vi "XYConstantCurr.vi"() -> ()   [LabVIEW 2014]
uses:
  <vilib>/Native 3D Graph/xcontrol/3DPC_SurfacePlot.xctl
  <vilib>/Instr/_visa.llb/VISA Configure Serial Port (Instr).vi
panel:
  out "XZ Graph":cluster{dbl[], dbl[]}(graph)
  in  "ScanStop":bool
  in  "STM Modefier":bool
  in  "LimitBeyondNum":i32
  out "Counting":i32(graph)
  out "ApprStop?":bool
  out "ZValue":dbl[](array[numeric])
  out "ProcRefCurr":dbl
  out "RMOVERR?":string
  out "XYPOS":cluster{dbl[], dbl[]}(graph)
  out "PIZPOSDia":dbl(graph)
  in  "ApproachStop":bool
  out "PIZERR? 2":string
  out "PIZERR?":string
  out "PreCurrDia":dbl(graph)
  out "3D Graph":refnum<class "Base Datatype.lvclass">[](xcontrol)
  in  "Y init/um":dbl format="%#_13g"
  in  "X init/um":dbl format="%#_13g"
  out "RefCurr":dbl
  out "PresCurr":dbl
  in  "PointNumToFresRefCurr":i32
  in  "ColumnNum":i32
  in  "RowNum":i32
  in  "ProbeBrokenDownToRefCurr %":dbl
  in  "TolerantIntervalToRefCurr %":dbl
  in  "CurrDecline %":dbl
  in  "PIZApproachStep/um":dbl
  in  "PIZAdjustStep/um":dbl
  in  "RoughYStep/um":dbl
  in  "RoughXStep/um":dbl
  out "PIZPos":dbl
  out "RoughZPos":dbl
  out "RoughYPos":dbl
  out "RoughXPos":dbl
  out "Outleak":string
  in  "PIZ":refnum<visa-resource-name>
  in  "RoughXYZ":refnum<visa-resource-name>
  in  "Volt":refnum<visa-resource-name>
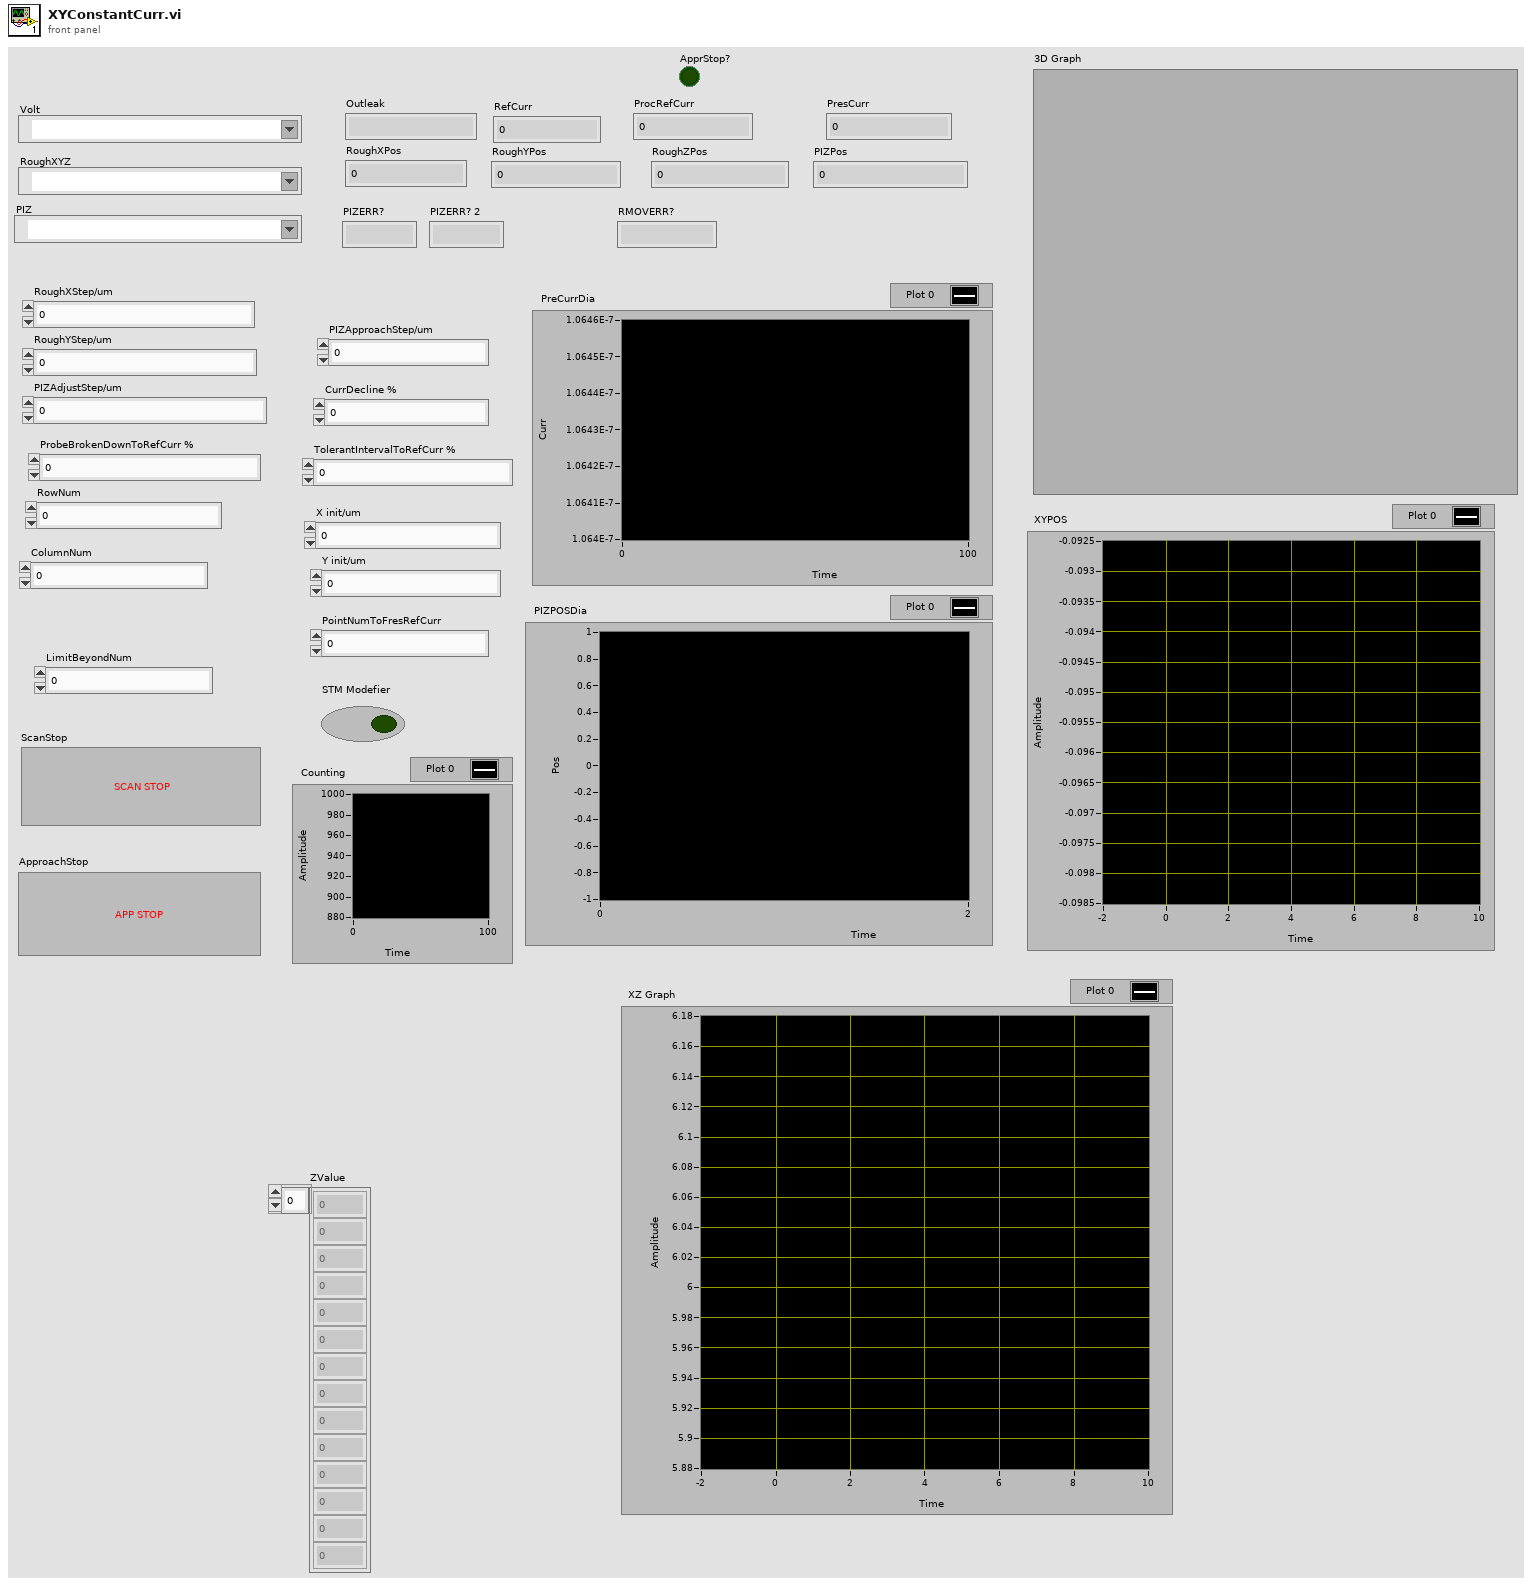
[diagram p1: front panel]
types:
  T1 = typedef "NI_Matrix.lvlib/RealMatrix.ctl" = dbl[][]
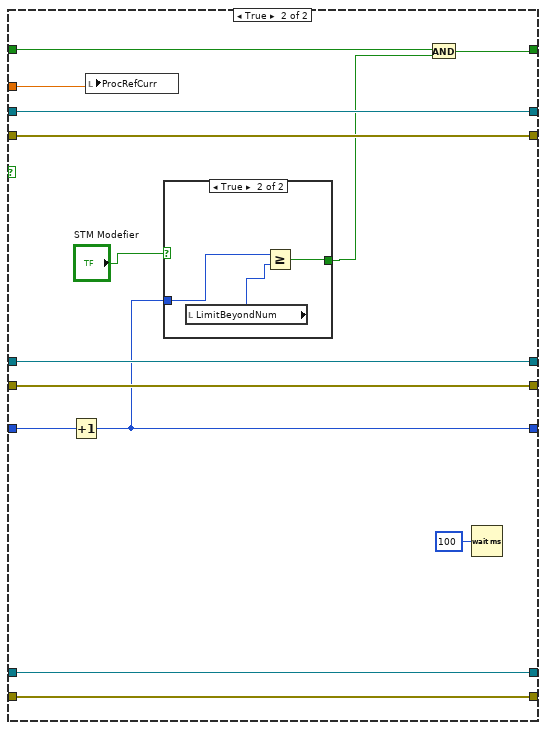
[diagram p2: hidden frame]
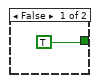
[diagram p3: hidden frame]
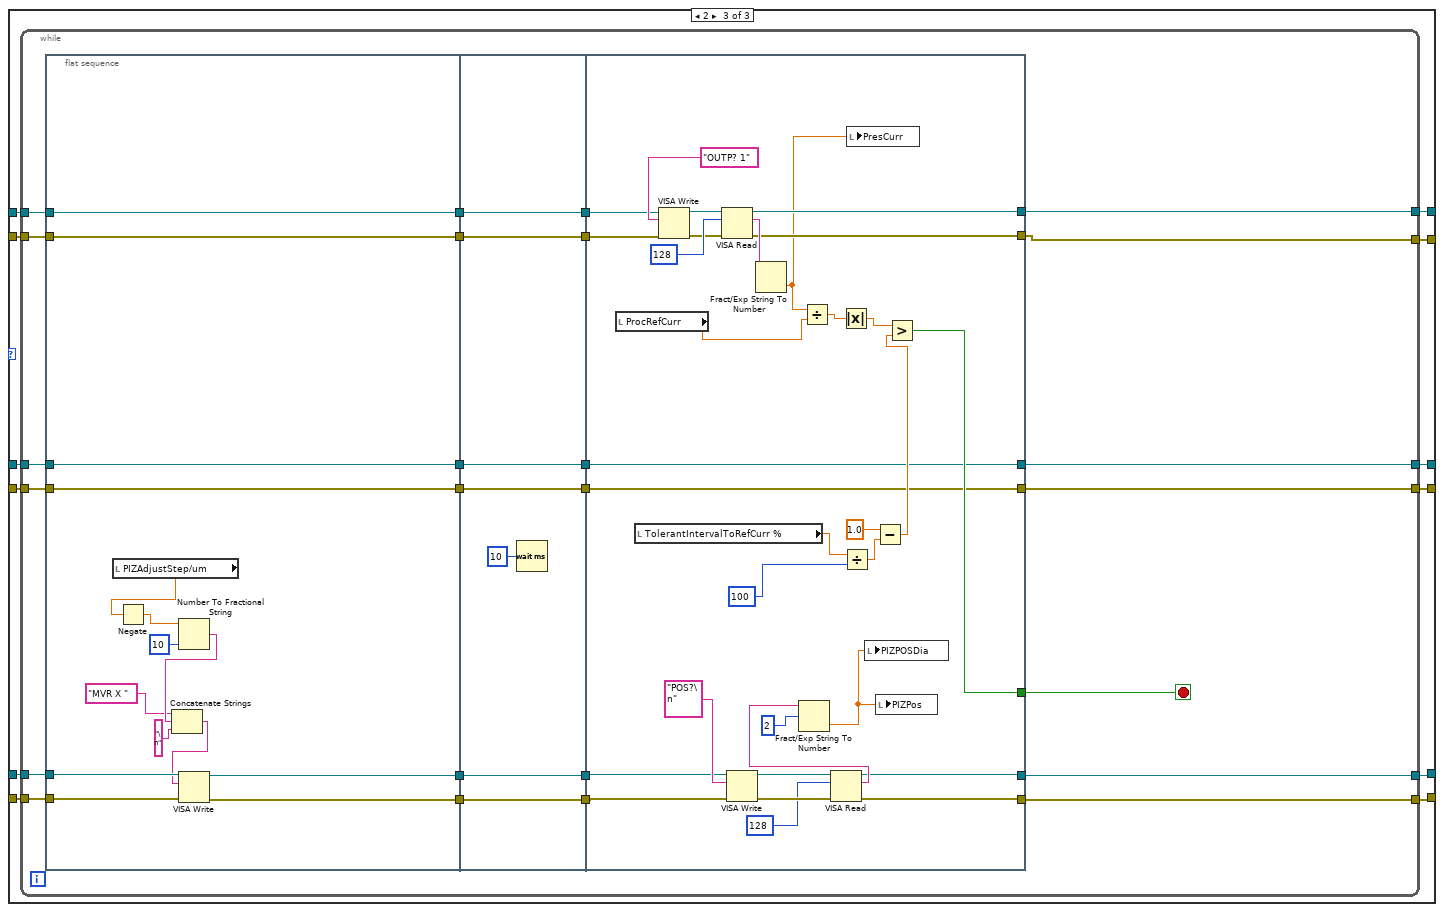
[diagram p5: hidden frame]
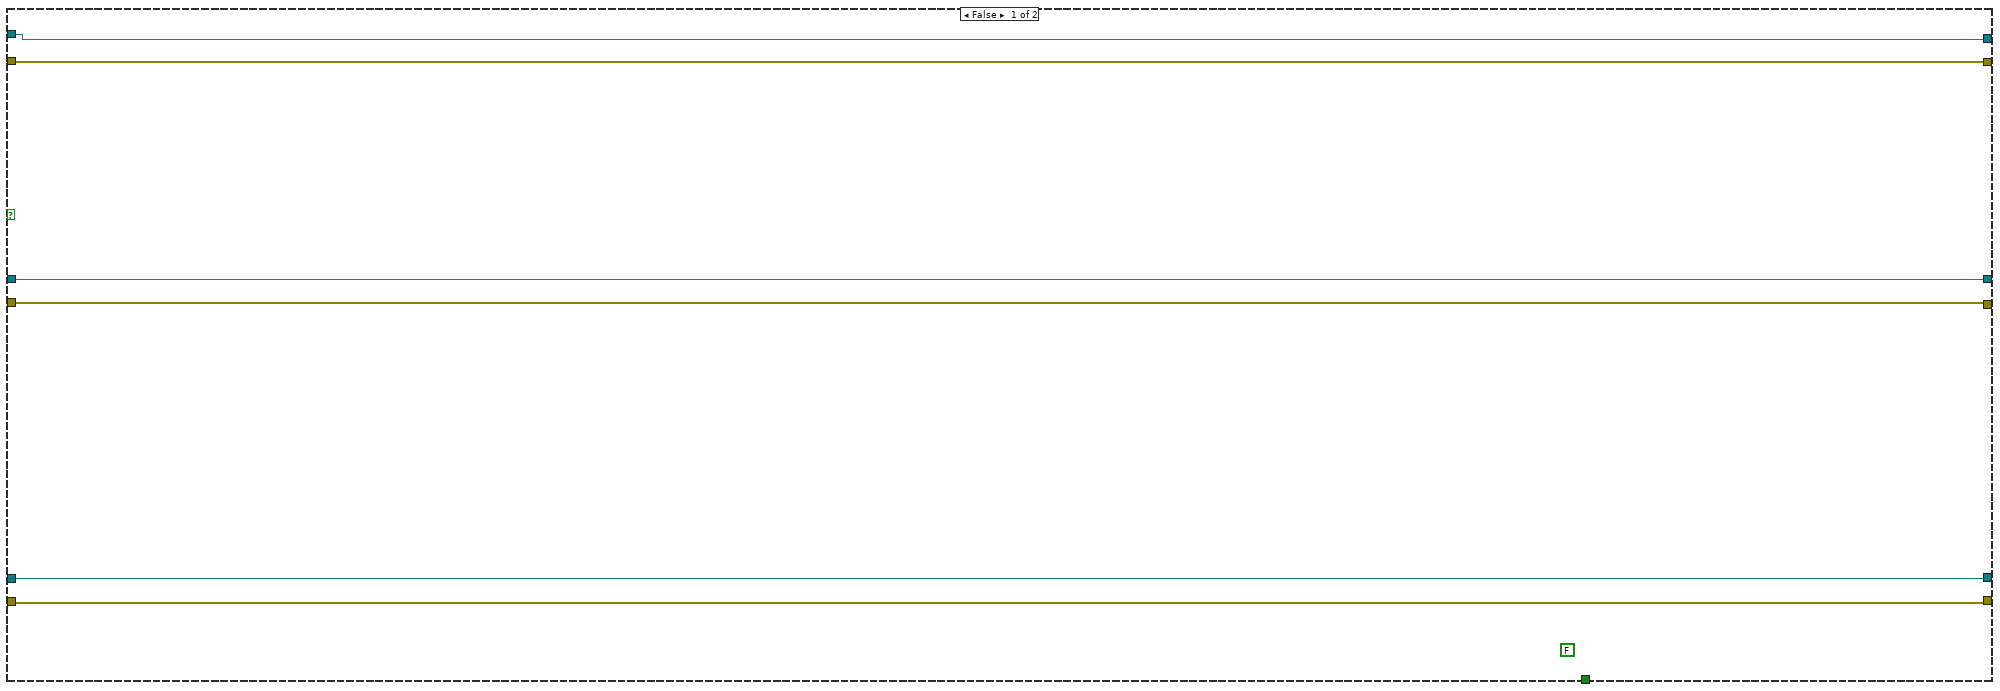
[diagram p6: hidden frame]
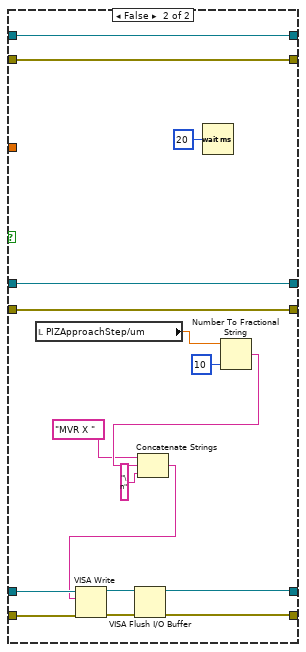
[diagram p8: hidden frame]
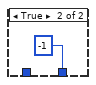
[diagram p10: hidden frame]
diagram:
  n1 = flat-sequence {
    tunnel: [w120] -> w82
    tunnel: [w119] -> w81
    tunnel: [w118] -> w80
    tunnel: [w117] -> w79
    tunnel: [w115] -> w78
    tunnel: [w114] -> w77
    tunnel: w82 -> [w185]
    tunnel: w81 -> [w184]
    tunnel: w80 -> [w169]
    tunnel: w79 -> [w168]
    tunnel: w78 -> [w193]
    tunnel: w77 -> [w192]
    tunnel: [w140] -> w76
    tunnel: [w139] -> w75
    tunnel: [w173] -> w74
    tunnel: [w172] -> w73
    tunnel: [w130] -> w72
    tunnel: [w129] -> w71
    tunnel: [w138] -> w66
    tunnel: w76 -> [w199]
    tunnel: w75 -> [w198]
    tunnel: w74 -> [w204]
    tunnel: w73 -> [w203]
    tunnel: w72 -> [w202]
    tunnel: w71 -> [w201]
    tunnel: [w204] -> w70
    tunnel: [w203] -> w69
    tunnel: [w202] -> w68
    tunnel: [w201] -> w67
    tunnel: w66 -> [w197]
    tunnel: [w194] -> w65
    tunnel: [w196] -> w64
    tunnel: [w195] -> w63
    tunnel: w70 -> [w232]
    tunnel: w69 -> [w231]
    tunnel: w68 -> [w230]
    tunnel: w67 -> [w229]
    tunnel: w65 -> [w221]
    tunnel: w64 -> [w234]
    tunnel: w63 -> [w233]
    tunnel: [w227] -> w6
    tunnel: [w226] -> w8
    tunnel: [w225] -> w10
    tunnel: [w224] -> w12
    tunnel: [w223] -> w14
    tunnel: [w222] -> w16
    tunnel: w16 -> [w320]
    tunnel: [w320] -> w15
    tunnel: w14 -> [w319]
    tunnel: [w319] -> w13
    tunnel: w12 -> [w318]
    tunnel: [w318] -> w11
    tunnel: w10 -> [w317]
    tunnel: [w317] -> w9
    tunnel: w8 -> [w316]
    tunnel: [w316] -> w7
    tunnel: w6 -> [w315]
    tunnel: [w315] -> w5
    tunnel: w15 -> [w335]
    tunnel: w13 -> [w336]
    tunnel: w11 -> [w323]
    tunnel: w9 -> [w324]
    tunnel: w7 -> [w349]
    tunnel: w5 -> [w350]
    tunnel: [w347] -> w62
    tunnel: [w346] -> w61
    tunnel: [w345] -> w60
    tunnel: [w344] -> w59
    tunnel: [w343] -> w58
    tunnel: [w342] -> w57
    tunnel: [w341] -> w39
    tunnel: [w340] -> w38
    tunnel: [w339] -> w37
    tunnel: w62 -> [w1192]
    tunnel: w61 -> [w1191]
    tunnel: w60 -> [w1194]
    tunnel: w59 -> [w1193]
    tunnel: w58 -> [w1199]
    tunnel: w57 -> [w1198]
    tunnel: [w1197] -> w56
    tunnel: [w1196] -> w55
    tunnel: [w1195] -> w54
    tunnel: [w1194] -> w53
    tunnel: [w1193] -> w52
    tunnel: [w1192] -> w51
    tunnel: [w1191] -> w50
    tunnel: w39 -> [w1189]
    tunnel: w38 -> [w1190]
    tunnel: w37 -> [w1188]
    tunnel: [w1190] -> w36
    tunnel: [w1189] -> w35
    tunnel: [w1188] -> w34
    tunnel: w56 -> [w1207]
    tunnel: w55 -> [w1206]
    tunnel: w54 -> [_]
    tunnel: w53 -> [w1214]
    tunnel: w52 -> [w1213]
    tunnel: w51 -> [w1212]
    tunnel: w50 -> [w1211]
    tunnel: [w1214] -> w49
    tunnel: [w1213] -> w48
    tunnel: [w1207] -> w47
    tunnel: [w1206] -> w46
    tunnel: [w1212] -> w45
    tunnel: [w1211] -> w44
    tunnel: w36 -> [w1210]
    tunnel: w35 -> [w1209]
    tunnel: w34 -> [w1208]
    tunnel: [w1210] -> w33
    tunnel: [w1209] -> w32
    tunnel: [w1208] -> w31
    tunnel: w49 -> [w1230]
    tunnel: w48 -> [w1229]
    tunnel: [w1220] -> w25
    tunnel: w47 -> [w1222]
    tunnel: [w1219] -> w24
    tunnel: w46 -> [w1221]
    tunnel: [w1227] -> w41
    tunnel: [w1226] -> w40
    tunnel: w45 -> [w1224]
    tunnel: w44 -> [w1223]
    tunnel: [w1224] -> w43
    tunnel: [w1223] -> w42
    tunnel: w33 -> [w1217]
    tunnel: w32 -> [w1216]
    tunnel: w31 -> [w1215]
    tunnel: [w1217] -> w29
    tunnel: [w1216] -> w28
    tunnel: [w1215] -> w27
    frame #0 {
      n2 = Wait (ms)(milliseconds to wait=u32 2000) -> ()  [unwired: 1 out]
      n3 = call-poly "VISA Configure Serial Port"("VISA resource name"="PIZ", "baud rate (9600)"=u32 115200) -> ("VISA resource name out"=w101:refnum<visa-resource-name>, "error out"=w100:errorcluster)  [unwired: 12 in]
      n4 = local write "CurrDecline %"("CurrDecline %") -> ()
      n5 = local write "TolerantIntervalToRefCurr %"("TolerantIntervalToRefCurr %") -> ()
      n6 = local write "ColumnNum"("ColumnNum") -> ()
      n7 = call-poly "VISA Configure Serial Port"("VISA resource name"="RoughXYZ", "baud rate (9600)"=u32 115200) -> ("VISA resource name out"=w92:refnum<visa-resource-name>, "error out"=w91:errorcluster)  [unwired: 12 in]
      n8 = local write "LimitBeyondNum"("LimitBeyondNum") -> ()
      n9 = local write "RowNum"("RowNum") -> ()
      n10 = local write "RoughYStep/um"("RoughYStep/um") -> ()
      n11 = local write "RoughXStep/um"("RoughXStep/um") -> ()
      n12 = local write "X init/um"("X init/um") -> ()
      n13 = VISA Write(VISA resource name=w101, write buffer="ERR?\n", error in (no error)=w100) -> (VISA resource name out=w99:refnum<visa-resource-name>, error out=w98:errorcluster)  [unwired: 1 out]
      n14 = VISA Write(VISA resource name=w92, write buffer="ERR?\n", error in (no error)=w91) -> (VISA resource name out=w89:refnum<visa-resource-name>, error out=w88:errorcluster)  [unwired: 1 out]
      n15 = VISA Read(VISA resource name=w99, byte count=u32 128, error in (no error)=w98) -> (VISA resource name out=w97:refnum<visa-resource-name>, read buffer=→"PIZERR?":string, error out=w96:errorcluster)  [unwired: 1 out]
      n16 = VISA Read(VISA resource name=w89, byte count=u32 128, error in (no error)=w88) -> (VISA resource name out=w87:refnum<visa-resource-name>, read buffer=→"RMOVERR?":string, error out=w86:errorcluster)  [unwired: 1 out]
      n17 = VISA Open(VISA resource name="Volt") -> (VISA resource name=w115:refnum<visa-resource-name>, error out=w114:errorcluster)  [unwired: 4 in]
      n18 = local write "PointNumToFresRefCurr"("PointNumToFresRefCurr") -> ()
      n19 = local write "ProbeBrokenDownToRefCurr %"("ProbeBrokenDownToRefCurr %") -> ()
      n20 = local write "PIZApproachStep/um"("PIZApproachStep/um") -> ()
      n21 = local write "PIZAdjustStep/um"("PIZAdjustStep/um") -> ()
      n22 = local write "Y init/um"("Y init/um") -> ()
      n23 = VISA Write(VISA resource name=w87, write buffer="ONL 1 1 2 1 3 1\nSVO A 1\nSVO B 1\nSVO C 1\n", error in (no error)=w86) -> (VISA resource name out=w120:refnum<visa-resource-name>, error out=w119:errorcluster)  [unwired: 1 out]
      n24 = VISA Write(VISA resource name=w97, write buffer="SVO X 1\n", error in (no error)=w96) -> (VISA resource name out=w118:refnum<visa-resource-name>, error out=w117:errorcluster)  [unwired: 1 out]
    }
    frame #1 {
      n25 = VISA Write(VISA resource name=w185, write buffer="POS? A\n", error in (no error)=w184) -> (VISA resource name out=w183:refnum<visa-resource-name>, error out=w182:errorcluster)  [unwired: 1 out]
      n26 = VISA Write(VISA resource name=w193, write buffer="OUTP? 1", error in (no error)=w192) -> (VISA resource name out=w190:refnum<visa-resource-name>, error out=w189:errorcluster)  [unwired: 1 out]
      n27 = VISA Write(VISA resource name=w169, write buffer="POS?\n", error in (no error)=w168) -> (VISA resource name out=w171:refnum<visa-resource-name>, error out=w170:errorcluster)  [unwired: 1 out]
      n28 = VISA Read(VISA resource name=w183, byte count=u32 128, error in (no error)=w182) -> (VISA resource name out=w181:refnum<visa-resource-name>, read buffer=w161:string, error out=w180:errorcluster)  [unwired: 1 out]
      n29 = VISA Read(VISA resource name=w190, byte count=u32 128, error in (no error)=w189) -> (VISA resource name out=w142:refnum<visa-resource-name>, read buffer=→"Outleak":string, error out=w141:errorcluster)  [unwired: 1 out]
      n30 = Fract/Exp String To Number(string=w161, offset=2) -> (number=→"RoughXPos":dbl)  [unwired: 2 in, 1 out]
      n31 = VISA Write(VISA resource name=w181, write buffer="POS? B\n", error in (no error)=w180) -> (VISA resource name out=w179:refnum<visa-resource-name>, error out=w178:errorcluster)  [unwired: 1 out]
      n32 = VISA Read(VISA resource name=w171, byte count=u32 128, error in (no error)=w170) -> (VISA resource name out=w132:refnum<visa-resource-name>, read buffer=w150:string, error out=w131:errorcluster)  [unwired: 1 out]
      n33 = VISA Read(VISA resource name=w179, byte count=u32 128, error in (no error)=w178) -> (VISA resource name out=w175:refnum<visa-resource-name>, read buffer=w160:string, error out=w174:errorcluster)  [unwired: 1 out]
      n34 = Fract/Exp String To Number(string=w150, offset=2) -> (number=→"PIZPos":dbl)  [unwired: 2 in, 1 out]
      n35 = Fract/Exp String To Number(string=w160, offset=2) -> (number=→"RoughYPos":dbl)  [unwired: 2 in, 1 out]
      n36 = VISA Write(VISA resource name=w132, write buffer="ERR?\n", error in (no error)=w131) -> (VISA resource name out=w137:refnum<visa-resource-name>, error out=w136:errorcluster)  [unwired: 1 out]
      n37 = VISA Write(VISA resource name=w142, write buffer="OUTP? 1", error in (no error)=w141) -> (VISA resource name out=w147:refnum<visa-resource-name>, error out=w146:errorcluster)  [unwired: 1 out]
      n38 = VISA Write(VISA resource name=w175, write buffer="POS? C\n", error in (no error)=w174) -> (VISA resource name out=w177:refnum<visa-resource-name>, error out=w176:errorcluster)  [unwired: 1 out]
      n39 = VISA Read(VISA resource name=w137, byte count=u32 128, error in (no error)=w136) -> (VISA resource name out=w130:refnum<visa-resource-name>, read buffer=→"PIZERR? 2":string, error out=w129:errorcluster)  [unwired: 1 out]
      n40 = VISA Read(VISA resource name=w177, byte count=u32 128, error in (no error)=w176) -> (VISA resource name out=w173:refnum<visa-resource-name>, read buffer=w159:string, error out=w172:errorcluster)  [unwired: 1 out]
      n41 = VISA Read(VISA resource name=w147, byte count=u32 128, error in (no error)=w146) -> (VISA resource name out=w140:refnum<visa-resource-name>, read buffer=w143:string, error out=w139:errorcluster)  [unwired: 1 out]
      n42 = Wait (ms)(milliseconds to wait=u32 1000) -> ()  [unwired: 1 out]
      n43 = Fract/Exp String To Number(string=w159, offset=2) -> (number=→"RoughZPos":dbl)  [unwired: 2 in, 1 out]
      n44 = Fract/Exp String To Number(string=w143) -> (number=w138:dbl)  [unwired: 3 in, 1 out]
      "ProcRefCurr" <- 0.0
    }
    frame #2 {
      # "Reference Curr"
      n45 = for {
        N: 50 -> [_]
        tunnel: w199 -> [w216]
        tunnel: w198 -> [w215]
        tunnel: [w213] -> w196
        tunnel: [w212] -> w195
        shift-right: [w207] -> w194
        shift-left: w197 -> [w210]
        n46 = VISA Write(VISA resource name=w216, write buffer="OUTP? 1", error in (no error)=w215) -> (VISA resource name out=w219:refnum<visa-resource-name>, error out=w218:errorcluster)  [unwired: 1 out]
        n47 = VISA Read(VISA resource name=w219, byte count=u32 128, error in (no error)=w218) -> (VISA resource name out=w213:refnum<visa-resource-name>, read buffer=w211:string, error out=w212:errorcluster)  [unwired: 1 out]
        n48 = Wait (ms)(milliseconds to wait=u32 1) -> ()  [unwired: 1 out]
        n49 = Fract/Exp String To Number(string=w211) -> (number=w205:dbl)  [unwired: 3 in, 1 out]
        "PresCurr" <- w205
        n50 = Add(x=w205, y=w210) -> (x+y=w209:dbl)
        n51 = Divide(x=w209, y=2.0) -> (x/y=w207:dbl)
      }
      "RefCurr" <- w194
    }
    frame #3 {
      n52 = local read "PIZApproachStep/um"() -> (w228:dbl)
      n53 = Divide(x=30.0, y=w228) -> (x/y=w236:dbl)
      n54 = Round Toward -Infinity(1:w236) -> (0:w235:dbl)
      n55 = for {
        N: w235 -> [_]
        tunnel: w234 -> [w274]
        tunnel: w233 -> [w273]
        tunnel: w232 -> [w270]
        tunnel: w231 -> [w269]
        tunnel: w230 -> [w255]
        tunnel: w229 -> [w254]
        tunnel: [w266] -> w227
        tunnel: [w265] -> w226
        tunnel: [w264] -> w225
        tunnel: [w263] -> w224
        tunnel: [w262] -> w223
        tunnel: [w261] -> w222
        tunnel: w221 -> [w250]
        shift-right: [w238] -> _
        shift-left: 0 -> [w239]
        stop <- w241 stop-if-true
        n56 = VISA Write(VISA resource name=w274, write buffer="OUTP? 1", error in (no error)=w273) -> (VISA resource name out=w279:refnum<visa-resource-name>, error out=w278:errorcluster)  [unwired: 1 out]
        n57 = VISA Write(VISA resource name=w255, write buffer="POS?\n", error in (no error)=w254) -> (VISA resource name out=w260:refnum<visa-resource-name>, error out=w259:errorcluster)  [unwired: 1 out]
        n58 = VISA Read(VISA resource name=w279, byte count=u32 128, error in (no error)=w278) -> (VISA resource name out=w272:refnum<visa-resource-name>, read buffer=w275:string, error out=w271:errorcluster)  [unwired: 1 out]
        n59 = VISA Read(VISA resource name=w260, byte count=u32 128, error in (no error)=w259) -> (VISA resource name out=w253:refnum<visa-resource-name>, read buffer=w256:string, error out=w252:errorcluster)  [unwired: 1 out]
        n60 = Fract/Exp String To Number(string=w275) -> (number=w240:dbl)  [unwired: 3 in, 1 out]
        "PreCurrDia" <- w240
        n61 = local read "CurrDecline %"() -> (w245:dbl)
        n62 = Fract/Exp String To Number(string=w256, offset=2) -> (number=w247:dbl)  [unwired: 2 in, 1 out]
        "PIZPOSDia" <- w247
        n63 = Subtract(x=w240, y=w250) -> (x-y=w268:dbl)
        n64 = local write "PresCurr"(w240) -> ()
        n65 = Absolute Value(x=w268) -> (abs(x)=w267:dbl)
        n66 = Divide(x=w245, y=100.0) -> (x/y=w244:dbl)
        n67 = Divide(x=w267, y=w250) -> (x/y=w243:dbl)
        n68 = local write "PIZPos"(w247) -> ()
        n69 = Greater Or Equal?(x=w243, y=w244) -> (x >= y?=w249:bool)
        n70 = Or(x=w249, y="ApproachStop") -> (x .or. y?=w242:bool)
        n71 = case shown="False" w249 {
          tunnel: w272 -> [w284 w309]
          tunnel: w271 -> [w283 w308]
          tunnel: w270 -> [w286 w307]
          tunnel: w269 -> [w285 w306]
          tunnel: w253 -> [w295 w297]
          tunnel: w252 -> [w294 w296]
          tunnel: [w284 w309] -> w266
          tunnel: [w283 w308] -> w265
          tunnel: [w286 w307] -> w264
          tunnel: [w285 w306] -> w263
          tunnel: [w288 w297] -> w262
          tunnel: [w287 w296] -> w261
          tunnel: w240 -> [_ w304]
          tunnel: w242 -> [w281 w302]
          tunnel: [w281 w298] -> w241
          tunnel: w239 -> [w280 w303]
          tunnel: [w280 w299] -> w238
          frame False {
            n72 = local read "PIZApproachStep/um"() -> (w292:dbl)
            n73 = Number To Fractional String(number=w292) -> (F-format string=w291:string)  [unwired: 3 in]
            n74 = Concatenate Strings("MVR X " ("write buffer"), w291, "\n" ("string")) -> (w289:string)
            n75 = VISA Write(VISA resource name=w295, write buffer=w289, error in (no error)=w294) -> (VISA resource name out=w288:refnum<visa-resource-name>, error out=w287:errorcluster)  [unwired: 1 out]
            n76 = Wait (ms)(milliseconds to wait=u32 10) -> ()  [unwired: 1 out]
          }
          frame True {
            n77 = Increment(x=w303) -> (x+1=w299:i32)
            n78 = local write "ProcRefCurr"(w304) -> ()
            n79 = case shown="True" "STM Modefier" {
              tunnel: [TRUE w313] -> w301
              tunnel: w299 -> [_ w312]
              frame False {
              }
              frame True {
                n80 = local read "LimitBeyondNum"() -> (w311:i32)
                n81 = Greater Or Equal?(x=w312, y=w311) -> (x >= y?=w313:bool)
              }
            }
            n82 = And(x=w302, y=w301) -> (x .and. y?=w298:bool)
            n83 = Wait (ms)(milliseconds to wait=u32 100) -> ()  [unwired: 1 out]
          }
        }
        "ApprStop?" <- w241
      }
    }
    frame #4 {
      n84 = Wait (ms)(milliseconds to wait=u32 200) -> ()  [unwired: 1 out]
    }
    frame #5 {
      w338 = dbl[] []
      w348 = 0
      # "Direction"
      # "Column Index"
      # "Row Index"
      n85 = VISA Write(VISA resource name=w336, write buffer="POS?\n", error in (no error)=w335) -> (VISA resource name out=w333:refnum<visa-resource-name>, error out=w332:errorcluster)  [unwired: 1 out]
      n86 = VISA Write(VISA resource name=w324, write buffer="ERR?\n", error in (no error)=w323) -> (VISA resource name out=w327:refnum<visa-resource-name>, error out=w326:errorcluster)  [unwired: 1 out]
      n87 = VISA Read(VISA resource name=w333, byte count=u32 128, error in (no error)=w332) -> (VISA resource name out=w331:refnum<visa-resource-name>, error out=w330:errorcluster)  [unwired: 2 out]
      n88 = VISA Read(VISA resource name=w327, byte count=u32 128, error in (no error)=w326) -> (VISA resource name out=w322:refnum<visa-resource-name>, error out=w321:errorcluster)  [unwired: 2 out]
      n89 = while {
        tunnel: w350 -> [w508]
        tunnel: w349 -> [w507]
        tunnel: w322 -> [w506]
        tunnel: w321 -> [w505]
        tunnel: w331 -> [w504]
        tunnel: w330 -> [w503]
        shift-right: [w442] -> _
        shift-left: 1 -> [w441]
        shift-right: [w438] -> _
        shift-left: w348 -> [w435]
        shift-right: [w437] -> _
        shift-left: w348 -> [w434]
        tunnel: [w426] -> w347
        tunnel: [w417] -> w346
        tunnel: [w412] -> w345
        tunnel: [w411] -> w344
        tunnel: [w406] -> w343
        tunnel: [w401] -> w342
        shift-right: [w363] -> w340
        shift-left: w338 -> [w360]
        shift-right: [w362] -> w341
        shift-left: w338 -> [w359]
        shift-right: [w361] -> w339
        shift-left: w338 -> [w358]
        i -> [w357]
        stop <- w436 stop-if-true
        n90 = flat-sequence {
          tunnel: w508 -> [w538]
          tunnel: w507 -> [w537]
          tunnel: w506 -> [w542]
          tunnel: w505 -> [w541]
          tunnel: w504 -> [w523]
          tunnel: w503 -> [w522]
          tunnel: [w538] -> w502
          tunnel: [w537] -> w501
          tunnel: [w526] -> w500
          tunnel: [w525] -> w499
          tunnel: [w523] -> w494
          tunnel: [w522] -> w493
          tunnel: w434 -> [w512]
          tunnel: w435 -> [w513]
          tunnel: [w513] -> w465
          tunnel: [w512] -> w464
          tunnel: w360 -> [w510]
          tunnel: w359 -> [w509]
          tunnel: [w511] -> w396
          tunnel: w358 -> [w511]
          tunnel: [w509] -> w394
          tunnel: [w510] -> w392
          tunnel: w502 -> [w553]
          tunnel: w501 -> [w552]
          tunnel: w500 -> [w551]
          tunnel: w499 -> [w550]
          tunnel: [w553] -> w498
          tunnel: [w552] -> w497
          tunnel: [w551] -> w496
          tunnel: [w550] -> w495
          tunnel: w494 -> [w549]
          tunnel: w493 -> [w548]
          tunnel: [w549] -> w492
          tunnel: [w548] -> w491
          tunnel: w465 -> [w547]
          tunnel: w464 -> [w546]
          tunnel: [w547] -> w462
          tunnel: [w546] -> w460
          tunnel: w396 -> [w545]
          tunnel: [w545] -> w395
          tunnel: w394 -> [w544]
          tunnel: [w544] -> w393
          tunnel: w392 -> [w543]
          tunnel: [w543] -> w391
          tunnel: w498 -> [w589]
          tunnel: w497 -> [w588]
          tunnel: w496 -> [w570]
          tunnel: w495 -> [w569]
          tunnel: w492 -> [w568]
          tunnel: w491 -> [w567]
          tunnel: [w582] -> w490
          tunnel: [w581] -> w489
          tunnel: [w570] -> w488
          tunnel: [w569] -> w487
          tunnel: [w568] -> w486
          tunnel: [w567] -> w485
          tunnel: [w564] -> w484
          tunnel: [w563] -> w463
          tunnel: w462 -> [w563]
          tunnel: [w562] -> w461
          tunnel: w460 -> [w562]
          tunnel: w395 -> [w559]
          tunnel: w393 -> [w560]
          tunnel: w391 -> [w561]
          tunnel: [w561] -> w390
          tunnel: [w560] -> w389
          tunnel: [w559] -> w382
          tunnel: w490 -> [w606]
          tunnel: w489 -> [w605]
          tunnel: w488 -> [w604]
          tunnel: w487 -> [w603]
          tunnel: w486 -> [w602]
          tunnel: w485 -> [w601]
          tunnel: w484 -> [w607]
          tunnel: [w600] -> w477
          tunnel: [w599] -> w475
          tunnel: [w598] -> w473
          tunnel: [w597] -> w471
          tunnel: [w596] -> w469
          tunnel: [w595] -> w467
          tunnel: w463 -> [w594]
          tunnel: w461 -> [w593]
          tunnel: [w594] -> w459
          tunnel: [w593] -> w458
          tunnel: w390 -> [w592]
          tunnel: w389 -> [w591]
          tunnel: [w592] -> w388
          tunnel: [w591] -> w386
          tunnel: [w590] -> w383
          tunnel: w382 -> [w590]
          tunnel: w477 -> [w820]
          tunnel: [w820] -> w476
          tunnel: w475 -> [w819]
          tunnel: [w819] -> w474
          tunnel: w473 -> [w818]
          tunnel: [w818] -> w472
          tunnel: w471 -> [w817]
          tunnel: [w817] -> w470
          tunnel: w469 -> [w816]
          tunnel: [w816] -> w468
          tunnel: w467 -> [w815]
          tunnel: [w815] -> w466
          tunnel: w459 -> [w813]
          tunnel: w458 -> [w812]
          tunnel: [w813] -> w457
          tunnel: [w812] -> w456
          tunnel: w388 -> [w810]
          tunnel: [w811] -> w387
          tunnel: w386 -> [w811]
          tunnel: [w810] -> w385
          tunnel: [w809] -> w384
          tunnel: w383 -> [w809]
          tunnel: w476 -> [w835]
          tunnel: [w833] -> w483
          tunnel: w474 -> [w834]
          tunnel: [w832] -> w482
          tunnel: w472 -> [w855]
          tunnel: [w847] -> w481
          tunnel: w470 -> [w854]
          tunnel: [w846] -> w480
          tunnel: w468 -> [w861]
          tunnel: [w861] -> w479
          tunnel: w466 -> [w860]
          tunnel: [w860] -> w478
          tunnel: w457 -> [w831]
          tunnel: w456 -> [w830]
          tunnel: [w831] -> w455
          tunnel: [w830] -> w454
          tunnel: w387 -> [w828]
          tunnel: w385 -> [w829]
          tunnel: w384 -> [w823]
          tunnel: [w825] -> w381
          tunnel: [w824] -> w380
          tunnel: [w822] -> w379
          tunnel: w357 -> [w873]
          tunnel: w483 -> [w893]
          tunnel: w482 -> [w892]
          tunnel: w481 -> [w891]
          tunnel: w480 -> [w890]
          tunnel: w479 -> [w889]
          tunnel: w478 -> [w888]
          tunnel: w455 -> [w887]
          tunnel: w454 -> [w886]
          tunnel: [w887] -> w453
          tunnel: [w886] -> w452
          tunnel: [w885] -> w433
          tunnel: [w884] -> w432
          tunnel: [w883] -> w431
          tunnel: [w882] -> w430
          tunnel: [w881] -> w429
          tunnel: [w880] -> w428
          tunnel: w381 -> [w876]
          tunnel: w380 -> [w879]
          tunnel: w379 -> [w875]
          tunnel: [w876] -> w377
          tunnel: [w879] -> w375
          tunnel: [w875] -> w374
          tunnel: ["ScanStop"] -> w356
          tunnel: w452 -> [w1090]
          tunnel: w453 -> [w1091]
          tunnel: w441 -> [w1088]
          tunnel: [w1087] -> w451
          tunnel: [w1086] -> w450
          tunnel: [w1085] -> w449
          tunnel: [w1083] -> w448
          tunnel: w433 -> [w1082]
          tunnel: w432 -> [w1081]
          tunnel: w431 -> [w1080]
          tunnel: w430 -> [w1079]
          tunnel: w429 -> [w1078]
          tunnel: w428 -> [w1077]
          tunnel: [w1082] -> w422
          tunnel: [w1081] -> w421
          tunnel: [w1080] -> w413
          tunnel: [w1079] -> w407
          tunnel: [w1078] -> w402
          tunnel: [w1077] -> w397
          tunnel: [w1076] -> w378
          tunnel: w377 -> [w1076]
          tunnel: [w1075] -> w376
          tunnel: w375 -> [w1075]
          tunnel: w374 -> [w1074]
          tunnel: [w1074] -> w370
          tunnel: w356 -> [w1073]
          tunnel: [w1073] -> w352
          tunnel: w451 -> [w1115]
          tunnel: w450 -> [w1120]
          tunnel: w449 -> [w1105]
          tunnel: w448 -> [w1116]
          tunnel: [w1117] -> w445
          tunnel: [w1119] -> w447
          tunnel: [w1118] -> w446
          tunnel: [w1114] -> w423
          tunnel: w422 -> [w1114]
          tunnel: w421 -> [w1113]
          tunnel: [w1113] -> w418
          tunnel: [w1112] -> w414
          tunnel: w413 -> [w1112]
          tunnel: [w1111] -> w408
          tunnel: w407 -> [w1111]
          tunnel: [w1110] -> w403
          tunnel: w402 -> [w1110]
          tunnel: [w1109] -> w398
          tunnel: w397 -> [w1109]
          tunnel: w378 -> [w1106]
          tunnel: w376 -> [w1107]
          tunnel: [w1108] -> w371
          tunnel: w370 -> [w1108]
          tunnel: [w1107] -> w367
          tunnel: [w1106] -> w364
          tunnel: [w1104] -> w353
          tunnel: w352 -> [w1104]
          tunnel: w447 -> [w1146]
          tunnel: w446 -> [w1133]
          tunnel: w445 -> [w1148]
          tunnel: [w1145] -> w444
          tunnel: [w1144] -> w443
          tunnel: [w1143] -> w442
          tunnel: [w1142] -> w424
          tunnel: w423 -> [w1142]
          tunnel: [w1141] -> w419
          tunnel: w418 -> [w1141]
          tunnel: [w1140] -> w415
          tunnel: w414 -> [w1140]
          tunnel: [w1139] -> w409
          tunnel: w408 -> [w1139]
          tunnel: [w1138] -> w404
          tunnel: w403 -> [w1138]
          tunnel: [w1137] -> w399
          tunnel: w398 -> [w1137]
          tunnel: [w1136] -> w372
          tunnel: w371 -> [w1136]
          tunnel: [w1135] -> w368
          tunnel: w367 -> [w1135]
          tunnel: [w1134] -> w365
          tunnel: w364 -> [w1134]
          tunnel: [w1132] -> w354
          tunnel: w353 -> [w1132]
          tunnel: w444 -> [w1172]
          tunnel: w443 -> [w1173]
          tunnel: w442 -> [w1171]
          tunnel: [w1172] -> w440
          tunnel: [w1170] -> w439
          tunnel: [w1169] -> w425
          tunnel: w424 -> [w1169]
          tunnel: [w1168] -> w420
          tunnel: w419 -> [w1168]
          tunnel: [w1167] -> w416
          tunnel: w415 -> [w1167]
          tunnel: [w1166] -> w410
          tunnel: w409 -> [w1166]
          tunnel: [w1165] -> w405
          tunnel: w404 -> [w1165]
          tunnel: [w1164] -> w400
          tunnel: w399 -> [w1164]
          tunnel: [w1163] -> w373
          tunnel: w372 -> [w1163]
          tunnel: [w1162] -> w369
          tunnel: w368 -> [w1162]
          tunnel: [w1161] -> w366
          tunnel: w365 -> [w1161]
          tunnel: [w1160] -> w355
          tunnel: w354 -> [w1160]
          tunnel: w440 -> [w1186]
          tunnel: w439 -> [w1187]
          tunnel: [w1186] -> w438
          tunnel: [w1187] -> w437
          tunnel: [w1184] -> w427
          tunnel: [w1183] -> w426
          tunnel: w425 -> [w1183]
          tunnel: [w1182] -> w417
          tunnel: w420 -> [w1182]
          tunnel: [w1181] -> w412
          tunnel: w416 -> [w1181]
          tunnel: [w1180] -> w411
          tunnel: w410 -> [w1180]
          tunnel: [w1179] -> w406
          tunnel: w405 -> [w1179]
          tunnel: [w1178] -> w401
          tunnel: w400 -> [w1178]
          tunnel: w373 -> [w1175]
          tunnel: w369 -> [w1176]
          tunnel: w366 -> [w1177]
          tunnel: [w1177] -> w363
          tunnel: [w1176] -> w362
          tunnel: [w1175] -> w361
          tunnel: [w1174] -> w351
          tunnel: w355 -> [w1174]
          frame #0 {
            n91 = local read "X init/um"() -> (w521:dbl)
            n92 = local read "RoughXStep/um"() -> (w519:dbl)
            n93 = Multiply(x=w519, y=w512) -> (x*y=w520:dbl)
            n94 = Add(x=w520, y=w521) -> (x+y=w518:dbl)
            n95 = Number To Fractional String(number=w518, precision (6)=i16 10) -> (F-format string=w533:string)  [unwired: 2 in]
            n96 = Concatenate Strings("MOV A " ("string"), w533, "\n" ("string")) -> (w528:string)
            n97 = VISA Write(VISA resource name=w542, write buffer=w528, error in (no error)=w541) -> (VISA resource name out=w540:refnum<visa-resource-name>, error out=w539:errorcluster)  [unwired: 1 out]
            n98 = local read "Y init/um"() -> (w516:dbl)
            n99 = local read "RoughYStep/um"() -> (w515:dbl)
            n100 = Wait (ms)(milliseconds to wait=u32 60) -> ()  [unwired: 1 out]
            n101 = Multiply(x=w515, y=w513) -> (x*y=w517:dbl)
            n102 = Add(x=w517, y=w516) -> (x+y=w514:dbl)
            n103 = Number To Fractional String(number=w514, precision (6)=i16 10) -> (F-format string=w534:string)  [unwired: 2 in]
            n104 = Concatenate Strings("MOV B " ("string"), w534, "\n" ("string")) -> (w527:string)
            n105 = VISA Write(VISA resource name=w540, write buffer=w527, error in (no error)=w539) -> (VISA resource name out=w526:refnum<visa-resource-name>, error out=w525:errorcluster)  [unwired: 1 out]
            "ZValue" <- w511
          }
          frame #1 {
            n106 = Wait (ms)(milliseconds to wait=u32 50) -> ()  [unwired: 1 out]
          }
          frame #2 {
            w578 = 1
            n107 = local read "TolerantIntervalToRefCurr %"() -> (w580:dbl)
            n108 = local read "ProcRefCurr"() -> (w557:dbl)
            n109 = VISA Write(VISA resource name=w589, write buffer="OUTP? 1", error in (no error)=w588) -> (VISA resource name out=w586:refnum<visa-resource-name>, error out=w585:errorcluster)  [unwired: 1 out]
            n110 = VISA Read(VISA resource name=w586, byte count=u32 128, error in (no error)=w585) -> (VISA resource name out=w582:refnum<visa-resource-name>, read buffer=w583:string, error out=w581:errorcluster)  [unwired: 1 out]
            n111 = Fract/Exp String To Number(string=w583) -> (number=w558:dbl)  [unwired: 3 in, 1 out]
            n112 = local write "PresCurr"(w558) -> ()
            n113 = Divide(x=w580, y=100.0) -> (x/y=w577:dbl)
            n114 = Divide(x=w558, y=w557) -> (x/y=w556:dbl)
            n115 = local write "PreCurrDia"(w558) -> ()
            n116 = Subtract(x=w578, y=w577) -> (x-y=w576:dbl)
            n117 = Add(x=w578, y=w577) -> (x+y=w575:dbl)
            n118 = Absolute Value(x=w556) -> (abs(x)=w555:dbl)
            n119 = Greater Or Equal?(x=w555, y=w575) -> (x >= y?=w574:bool)
            n120 = Less Or Equal?(x=w555, y=w576) -> (x <= y?=w573:bool)
            n121 = Boolean To (0,1)(Boolean=w574) -> (0, 1=w565:i16)
            n122 = Boolean To (0,1)(Boolean=w573) -> (0, 1=w572:i16)
            n123 = Multiply(x=w572, y=i16 2) -> (x*y=w566:i16)
            n124 = Add(x=w565, y=w566) -> (x+y=w564:i16)
          }
          frame #3 {
            n125 = case shown="1" w607 {
              tunnel: w606 -> [w613 w625 w729]
              tunnel: w605 -> [w612 w624 w728]
              tunnel: w604 -> [w611 w623 w727]
              tunnel: w603 -> [w610 w622 w726]
              tunnel: w602 -> [w609 w621 w725]
              tunnel: w601 -> [w608 w620 w724]
              tunnel: [w611 w619 w721] -> w598
              tunnel: [w610 w618 w720] -> w597
              tunnel: [w613 w617 w723] -> w596
              tunnel: [w612 w616 w722] -> w595
              tunnel: [w609 w615 w719] -> w600
              tunnel: [w608 w614 w718] -> w599
              frame 0, Default {
              }
              frame 1 {
                n126 = while {
                  tunnel: w625 -> [w657]
                  tunnel: w624 -> [w656]
                  tunnel: w623 -> [w655]
                  tunnel: w622 -> [w654]
                  tunnel: w621 -> [w653]
                  tunnel: w620 -> [w652]
                  tunnel: [w639] -> w617
                  tunnel: [w636] -> w616
                  tunnel: [w633] -> w619
                  tunnel: [w632] -> w618
                  tunnel: [w629] -> w615
                  tunnel: [w628] -> w614
                  stop <- w626 stop-if-true
                  n127 = flat-sequence {
                    tunnel: w657 -> [w671]
                    tunnel: w656 -> [w670]
                    tunnel: w655 -> [w669]
                    tunnel: w654 -> [w668]
                    tunnel: w653 -> [w667]
                    tunnel: w652 -> [w666]
                    tunnel: [w671] -> w651
                    tunnel: [w670] -> w649
                    tunnel: [w669] -> w647
                    tunnel: [w668] -> w645
                    tunnel: [w660] -> w643
                    tunnel: [w659] -> w642
                    tunnel: w651 -> [w678]
                    tunnel: [w678] -> w650
                    tunnel: w649 -> [w677]
                    tunnel: [w677] -> w648
                    tunnel: w647 -> [w676]
                    tunnel: [w676] -> w646
                    tunnel: w645 -> [w675]
                    tunnel: [w675] -> w644
                    tunnel: w643 -> [w674]
                    tunnel: w642 -> [w673]
                    tunnel: [w674] -> w641
                    tunnel: [w673] -> w640
                    tunnel: w650 -> [w705]
                    tunnel: w648 -> [w704]
                    tunnel: w646 -> [w696]
                    tunnel: w644 -> [w695]
                    tunnel: w641 -> [w691]
                    tunnel: w640 -> [w690]
                    tunnel: [w698] -> w638
                    tunnel: [w697] -> w637
                    tunnel: [w696] -> w635
                    tunnel: [w695] -> w634
                    tunnel: [w687] -> w631
                    tunnel: [w686] -> w630
                    tunnel: [w692] -> w627
                    tunnel: [w717] -> w639
                    tunnel: w638 -> [w717]
                    tunnel: [w716] -> w636
                    tunnel: w637 -> [w716]
                    tunnel: w635 -> [w715]
                    tunnel: [w715] -> w633
                    tunnel: w634 -> [w714]
                    tunnel: [w714] -> w632
                    tunnel: w631 -> [w713]
                    tunnel: w630 -> [w712]
                    tunnel: [w713] -> w629
                    tunnel: [w712] -> w628
                    tunnel: [w711] -> w626
                    tunnel: w627 -> [w711]
                    frame #0 {
                      n128 = local read "PIZAdjustStep/um"() -> (w658:dbl)
                      n129 = Number To Fractional String(number=w658, precision (6)=i16 10) -> (F-format string=w663:string)  [unwired: 2 in]
                      n130 = Concatenate Strings("MVR X ", w663, "\n" ("string")) -> (w661:string)
                      n131 = VISA Write(VISA resource name=w667, write buffer=w661, error in (no error)=w666) -> (VISA resource name out=w660:refnum<visa-resource-name>, error out=w659:errorcluster)  [unwired: 1 out]
                    }
                    frame #1 {
                      n132 = Wait (ms)(milliseconds to wait=u32 10) -> ()  [unwired: 1 out]
                    }
                    frame #2 {
                      n133 = local read "TolerantIntervalToRefCurr %"() -> (w703:dbl)
                      n134 = local read "ProcRefCurr"() -> (w693:dbl)
                      n135 = VISA Write(VISA resource name=w705, write buffer="OUTP? 1", error in (no error)=w704) -> (VISA resource name out=w706:refnum<visa-resource-name>, error out=w707:errorcluster)  [unwired: 1 out]
                      n136 = VISA Write(VISA resource name=w691, write buffer="POS?\n", error in (no error)=w690) -> (VISA resource name out=w689:refnum<visa-resource-name>, error out=w688:errorcluster)  [unwired: 1 out]
                      n137 = VISA Read(VISA resource name=w706, byte count=u32 128, error in (no error)=w707) -> (VISA resource name out=w698:refnum<visa-resource-name>, read buffer=w709:string, error out=w697:errorcluster)  [unwired: 1 out]
                      n138 = Fract/Exp String To Number(string=w709) -> (number=w694:dbl)  [unwired: 3 in, 1 out]
                      n139 = Divide(x=w694, y=w693) -> (x/y=w680:dbl)
                      n140 = VISA Read(VISA resource name=w689, byte count=u32 128, error in (no error)=w688) -> (VISA resource name out=w687:refnum<visa-resource-name>, read buffer=w683:string, error out=w686:errorcluster)  [unwired: 1 out]
                      n141 = local write "PresCurr"(w694) -> ()
                      n142 = Divide(x=w703, y=100.0) -> (x/y=w700:dbl)
                      n143 = Fract/Exp String To Number(string=w683, offset=2) -> (number=w681:dbl)  [unwired: 2 in, 1 out]
                      n144 = Absolute Value(x=w680) -> (abs(x)=w679:dbl)
                      n145 = Add(x=1, y=w700) -> (x+y=w699:dbl)
                      n146 = local write "PIZPOSDia"(w681) -> ()
                      n147 = local write "PreCurrDia"(w694) -> ()
                      n148 = local write "PIZPos"(w681) -> ()
                      n149 = Less?(x=w679, y=w699) -> (x < y?=w692:bool)
                    }
                    frame #3 {
                    }
                  }
                }
              }
              frame 2 {
                n150 = while {
                  tunnel: w729 -> [w750]
                  tunnel: w728 -> [w749]
                  tunnel: w727 -> [w748]
                  tunnel: w726 -> [w747]
                  tunnel: w725 -> [w746]
                  tunnel: w724 -> [w745]
                  tunnel: [w735] -> w723
                  tunnel: [w734] -> w722
                  tunnel: [w733] -> w721
                  tunnel: [w732] -> w720
                  tunnel: [w731] -> w719
                  tunnel: [w730] -> w718
                  stop <- w736 stop-if-true
                  n151 = flat-sequence {
                    tunnel: [w769] -> w754
                    tunnel: w750 -> [w769]
                    tunnel: [w768] -> w753
                    tunnel: w749 -> [w768]
                    tunnel: [w767] -> w752
                    tunnel: w748 -> [w767]
                    tunnel: [w766] -> w751
                    tunnel: w747 -> [w766]
                    tunnel: w746 -> [w764]
                    tunnel: w745 -> [w765]
                    tunnel: [w758] -> w744
                    tunnel: [w757] -> w743
                    tunnel: w754 -> [w776]
                    tunnel: w753 -> [w775]
                    tunnel: w752 -> [w774]
                    tunnel: w751 -> [w773]
                    tunnel: w744 -> [w772]
                    tunnel: w743 -> [w771]
                    tunnel: [w776] -> w742
                    tunnel: [w775] -> w741
                    tunnel: [w774] -> w740
                    tunnel: [w773] -> w739
                    tunnel: [w772] -> w738
                    tunnel: [w771] -> w737
                    tunnel: w742 -> [w803]
                    tunnel: w741 -> [w802]
                    tunnel: w740 -> [w792]
                    tunnel: w739 -> [w791]
                    tunnel: w738 -> [w783]
                    tunnel: w737 -> [w782]
                    tunnel: [w801] -> w735
                    tunnel: [w800] -> w734
                    tunnel: [w794] -> w736
                    tunnel: [w792] -> w733
                    tunnel: [w791] -> w732
                    tunnel: [w781] -> w731
                    tunnel: [w780] -> w730
                    frame #0 {
                      n152 = local read "PIZAdjustStep/um"() -> (w756:dbl)
                      n153 = Negate(x=w756) -> (-x=w755:dbl)
                      n154 = Number To Fractional String(number=w755, precision (6)=i16 10) -> (F-format string=w761:string)  [unwired: 2 in]
                      n155 = Concatenate Strings("MVR X " ("string"), w761, "\n" ("string")) -> (w763:string)
                      n156 = VISA Write(VISA resource name=w764, write buffer=w763, error in (no error)=w765) -> (VISA resource name out=w758:refnum<visa-resource-name>, error out=w757:errorcluster)  [unwired: 1 out]
                    }
                    frame #1 {
                      n157 = Wait (ms)(milliseconds to wait=u32 10) -> ()  [unwired: 1 out]
                    }
                    frame #2 {
                      n158 = local read "ProcRefCurr"() -> (w790:dbl)
                      n159 = local read "TolerantIntervalToRefCurr %"() -> (w798:dbl)
                      n160 = VISA Write(VISA resource name=w803, write buffer="OUTP? 1", error in (no error)=w802) -> (VISA resource name out=w804:refnum<visa-resource-name>, error out=w805:errorcluster)  [unwired: 1 out]
                      n161 = VISA Read(VISA resource name=w804, byte count=u32 128, error in (no error)=w805) -> (VISA resource name out=w801:refnum<visa-resource-name>, read buffer=w807:string, error out=w800:errorcluster)  [unwired: 1 out]
                      n162 = VISA Write(VISA resource name=w783, write buffer="POS?\n", error in (no error)=w782) -> (VISA resource name out=w789:refnum<visa-resource-name>, error out=w788:errorcluster)  [unwired: 1 out]
                      n163 = Fract/Exp String To Number(string=w807) -> (number=w799:dbl)  [unwired: 3 in, 1 out]
                      n164 = Divide(x=w799, y=w790) -> (x/y=w778:dbl)
                      n165 = VISA Read(VISA resource name=w789, byte count=u32 128, error in (no error)=w788) -> (VISA resource name out=w781:refnum<visa-resource-name>, read buffer=w785:string, error out=w780:errorcluster)  [unwired: 1 out]
                      n166 = Fract/Exp String To Number(string=w785, offset=2) -> (number=w779:dbl)  [unwired: 2 in, 1 out]
                      n167 = Absolute Value(x=w778) -> (abs(x)=w777:dbl)
                      n168 = Divide(x=w798, y=100) -> (x/y=w796:dbl)
                      n169 = local write "PresCurr"(w799) -> ()
                      n170 = local write "PIZPOSDia"(w779) -> ()
                      n171 = Subtract(x=1.0, y=w796) -> (x-y=w793:dbl)
                      n172 = local write "PIZPos"(w779) -> ()
                      n173 = Greater?(x=w777, y=w793) -> (0:w794:bool)
                    }
                  }
                }
              }
            }
          }
          frame #4 {
            n174 = Wait (ms)(milliseconds to wait=u32 10) -> ()  [unwired: 1 out]
          }
          frame #5 {
            n175 = VISA Write(VISA resource name=w855, write buffer="POS? A\n", error in (no error)=w854) -> (VISA resource name out=w856:refnum<visa-resource-name>, error out=w857:errorcluster)  [unwired: 1 out]
            n176 = VISA Read(VISA resource name=w856, byte count=u32 128, error in (no error)=w857) -> (VISA resource name out=w849:refnum<visa-resource-name>, read buffer=w859:string, error out=w848:errorcluster)  [unwired: 1 out]
            n177 = Fract/Exp String To Number(string=w859, offset=2) -> (number=w827:dbl)  [unwired: 2 in, 1 out]
            n178 = Build Array (concatenate)(w829, w827) -> (w825:dbl[])
            n179 = VISA Write(VISA resource name=w835, write buffer="POS? X\n", error in (no error)=w834) -> (VISA resource name out=w838:refnum<visa-resource-name>, error out=w839:errorcluster)  [unwired: 1 out]
            n180 = VISA Write(VISA resource name=w849, write buffer="POS? B\n", error in (no error)=w848) -> (VISA resource name out=w850:refnum<visa-resource-name>, error out=w851:errorcluster)  [unwired: 1 out]
            n181 = VISA Read(VISA resource name=w838, byte count=u32 128, error in (no error)=w839) -> (VISA resource name out=w833:refnum<visa-resource-name>, read buffer=w841:string, error out=w832:errorcluster)  [unwired: 1 out]
            n182 = VISA Read(VISA resource name=w850, byte count=u32 128, error in (no error)=w851) -> (VISA resource name out=w847:refnum<visa-resource-name>, read buffer=w853:string, error out=w846:errorcluster)  [unwired: 1 out]
            n183 = Fract/Exp String To Number(string=w841, offset=2) -> (number=w821:dbl)  [unwired: 2 in, 1 out]
            n184 = Build Array (concatenate)(w823, w821) -> (w822:dbl[])
            n185 = Fract/Exp String To Number(string=w853, offset=2) -> (number=w826:dbl)  [unwired: 2 in, 1 out]
            n186 = Build Array (concatenate)(w828, w826) -> (w824:dbl[])
            n187 = local write "PIZPOSDia"(w821) -> ()
          }
          frame #6 {
            n188 = local read "ProbeBrokenDownToRefCurr %"() -> (w864:dbl)
            n189 = local read "ProcRefCurr"() -> (w866:dbl)
            n190 = local read "PointNumToFresRefCurr"() -> (w871:i32)
            n191 = local read "PresCurr"() -> (w867:dbl)
            n192 = Quotient & Remainder(x=w873, y=w871) -> (x-y*floor(x/y)=w872:i32)  [unwired: 1 out]
            n193 = Decrement(x=w871) -> (x-1=w870:i32)
            n194 = Greater Or Equal?(x=w872, y=w870) -> (x >= y?=w868:bool)
            n195 = Subtract(x=w867, y=w866) -> (x-y=w862:dbl)
            n196 = Bundle(w876, w879) -> (→"XYPOS":cluster{dbl[], dbl[]})  [unwired: 1 in]
            n197 = Divide(x=w862, y=w866) -> (x/y=w865:dbl)
            n198 = Greater Or Equal?(x=w865, y=w864) -> (x >= y?=w863:bool)
            n199 = Or(x=w863, y=w868) -> (x .or. y?=w869:bool)
            n200 = case shown="True" w869 {
              tunnel: w893 -> [w896 w933]
              tunnel: w892 -> [w895 w932]
              tunnel: w891 -> [w897 w935]
              tunnel: w890 -> [w894 w934]
              tunnel: w889 -> [w899 w937]
              tunnel: w888 -> [w898 w936]
              tunnel: [w899 w908] -> w885
              tunnel: [w898 w907] -> w884
              tunnel: [w897 w906] -> w883
              tunnel: [w894 w905] -> w882
              tunnel: [w896 w904] -> w881
              tunnel: [w895 w903] -> w880
              tunnel: "ScanStop" -> [_ w902]
              frame False {
                (unwired) FALSE
              }
              frame True {
                n201 = flat-sequence {
                  tunnel: w937 -> [w941]
                  tunnel: w936 -> [w940]
                  tunnel: w935 -> [w943]
                  tunnel: w934 -> [w942]
                  tunnel: w933 -> [w951]
                  tunnel: w932 -> [w952]
                  tunnel: [w943] -> w931
                  tunnel: [w942] -> w930
                  tunnel: [w941] -> w929
                  tunnel: [w940] -> w928
                  tunnel: [w939] -> w901
                  tunnel: [w938] -> w900
                  tunnel: w931 -> [w961]
                  tunnel: w930 -> [w960]
                  tunnel: w929 -> [w959]
                  tunnel: w928 -> [w958]
                  tunnel: [w961] -> w927
                  tunnel: [w960] -> w926
                  tunnel: [w959] -> w925
                  tunnel: [w958] -> w924
                  tunnel: [w955] -> w922
                  tunnel: [w954] -> w920
                  tunnel: w901 -> [w957]
                  tunnel: w900 -> [w956]
                  tunnel: w927 -> [w964]
                  tunnel: w926 -> [w963]
                  tunnel: w925 -> [w966]
                  tunnel: w924 -> [w965]
                  tunnel: [w968] -> w923
                  tunnel: w922 -> [w968]
                  tunnel: [w967] -> w921
                  tunnel: w920 -> [w967]
                  tunnel: [w966] -> w919
                  tunnel: [w965] -> w918
                  tunnel: [w964] -> w917
                  tunnel: [w963] -> w916
                  tunnel: w923 -> [w971]
                  tunnel: w921 -> [w970]
                  tunnel: w919 -> [w979]
                  tunnel: w918 -> [w978]
                  tunnel: w917 -> [w975]
                  tunnel: w916 -> [w974]
                  tunnel: [w975] -> w915
                  tunnel: [w974] -> w914
                  tunnel: [w973] -> w913
                  tunnel: [w972] -> w912
                  tunnel: [w971] -> w911
                  tunnel: [w970] -> w910
                  tunnel: [w969] -> w909
                  tunnel: w915 -> [w1011]
                  tunnel: w914 -> [w1010]
                  tunnel: w913 -> [w1013]
                  tunnel: w912 -> [w1012]
                  tunnel: w911 -> [w1009]
                  tunnel: w910 -> [w1008]
                  tunnel: w909 -> [w1007]
                  tunnel: [w1006] -> w908
                  tunnel: [w1005] -> w907
                  tunnel: [w1004] -> w906
                  tunnel: [w1003] -> w905
                  tunnel: [w1002] -> w904
                  tunnel: [w1001] -> w903
                  tunnel: w902 -> [w1000]
                  frame #0 {
                    n202 = VISA Write(VISA resource name=w951, write buffer="POS?\n", error in (no error)=w952) -> (VISA resource name out=w950:refnum<visa-resource-name>, error out=w949:errorcluster)  [unwired: 1 out]
                    n203 = VISA Read(VISA resource name=w950, byte count=u32 128, error in (no error)=w949) -> (VISA resource name out=w939:refnum<visa-resource-name>, read buffer=w946:string, error out=w938:errorcluster)  [unwired: 1 out]
                    n204 = Fract/Exp String To Number(string=w946, offset=2) -> (number=w944:dbl)  [unwired: 2 in, 1 out]
                    n205 = local write "PIZPos"(w944) -> ()
                  }
                  frame #1 {
                    n206 = VISA Write(VISA resource name=w957, write buffer="MOV X 0\n" ("string"), error in (no error)=w956) -> (VISA resource name out=w955:refnum<visa-resource-name>, error out=w954:errorcluster)  [unwired: 1 out]
                  }
                  frame #2 {
                    n207 = Wait (ms)(milliseconds to wait=u32 10) -> ()  [unwired: 1 out]
                  }
                  frame #3 {
                    n208 = for {
                      N: 50 -> [_]
                      tunnel: w979 -> [w995]
                      tunnel: w978 -> [w994]
                      tunnel: [w989] -> w973
                      tunnel: [w988] -> w972
                      shift-right: [w980] -> w969
                      shift-left: 0.0 -> [w983]
                      i -> [w986]
                      n209 = VISA Write(VISA resource name=w995, write buffer="OUTP? 1", error in (no error)=w994) -> (VISA resource name out=w992:refnum<visa-resource-name>, error out=w991:errorcluster)  [unwired: 1 out]
                      n210 = Equal?(x=0, y=w986) -> (x = y?=w984:bool)
                      n211 = VISA Read(VISA resource name=w992, byte count=u32 128, error in (no error)=w991) -> (VISA resource name out=w989:refnum<visa-resource-name>, read buffer=w987:string, error out=w988:errorcluster)  [unwired: 1 out]
                      n212 = Fract/Exp String To Number(string=w987) -> (number=w982:dbl)  [unwired: 3 in, 1 out]
                      n213 = Add(x=w982, y=w983) -> (x+y=w981:dbl)
                      n214 = case shown="False" w984 {
                        tunnel: w981 -> [w998 w999]
                        tunnel: [w996 w999] -> w980
                        frame False {
                          n215 = Divide(x=w998, y=2.0) -> (x/y=w996:dbl)
                        }
                        frame True {
                        }
                      }
                    }
                    n216 = local write "RefCurr"(w969) -> ()
                  }
                  frame #4 {
                    n217 = local read "PIZApproachStep/um"() -> (w1016:dbl)
                    n218 = Divide(x=30.0, y=w1016) -> (x/y=w1015:dbl)
                    n219 = Round Toward -Infinity(1:w1015) -> (0:w1014:dbl)
                    n220 = for {
                      N: w1014 -> [_]
                      tunnel: w1013 -> [w1042]
                      tunnel: w1012 -> [w1041]
                      tunnel: w1011 -> [w1035]
                      tunnel: w1010 -> [w1034]
                      tunnel: w1009 -> [w1033]
                      tunnel: w1008 -> [w1032]
                      tunnel: w1007 -> [w1038]
                      tunnel: [w1031] -> w1006
                      tunnel: [w1030] -> w1005
                      tunnel: [w1029] -> w1004
                      tunnel: [w1028] -> w1003
                      tunnel: [w1027] -> w1002
                      tunnel: [w1026] -> w1001
                      tunnel: w1000 -> [w1018]
                      stop <- w1019 stop-if-true
                      n221 = local read "CurrDecline %"() -> (w1024:dbl)
                      n222 = VISA Write(VISA resource name=w1042, write buffer="OUTP? 1", error in (no error)=w1041) -> (VISA resource name out=w1046:refnum<visa-resource-name>, error out=w1045:errorcluster)  [unwired: 1 out]
                      n223 = VISA Read(VISA resource name=w1046, byte count=u32 128, error in (no error)=w1045) -> (VISA resource name out=w1037:refnum<visa-resource-name>, read buffer=w1043:string, error out=w1036:errorcluster)  [unwired: 1 out]
                      n224 = Fract/Exp String To Number(string=w1043) -> (number=w1021:dbl)  [unwired: 3 in, 1 out]
                      n225 = Subtract(x=w1021, y=w1038) -> (x-y=w1040:dbl)
                      n226 = Absolute Value(x=w1040) -> (abs(x)=w1039:dbl)
                      n227 = Divide(x=w1039, y=w1038) -> (x/y=w1025:dbl)
                      n228 = Divide(x=w1024, y=100.0) -> (x/y=w1022:dbl)
                      n229 = local write "PreCurrDia"(w1021) -> ()
                      n230 = local write "PresCurr"(w1021) -> ()
                      n231 = Greater Or Equal?(x=w1025, y=w1022) -> (x >= y?=w1020:bool)
                      n232 = Or(x=w1020, y=w1018) -> (x .or. y?=w1019:bool)
                      n233 = case shown="True" w1019 {
                        tunnel: w1037 -> [w1055 w1072]
                        tunnel: w1036 -> [w1054 w1071]
                        tunnel: w1035 -> [w1053 w1070]
                        tunnel: w1034 -> [w1052 w1069]
                        tunnel: w1033 -> [w1051 w1068]
                        tunnel: w1032 -> [w1050 w1067]
                        tunnel: [w1055 w1072] -> w1031
                        tunnel: [w1054 w1071] -> w1030
                        tunnel: [w1053 w1070] -> w1029
                        tunnel: [w1052 w1069] -> w1028
                        tunnel: [w1051 w1064] -> w1027
                        tunnel: [w1050 w1063] -> w1026
                        tunnel: w1021 -> [w1049 _]
                        frame True {
                          n234 = local write "ProcRefCurr"(w1049) -> ()
                          n235 = Wait (ms)(milliseconds to wait=u32 100) -> ()  [unwired: 1 out]
                        }
                        frame False {
                          n236 = local read "PIZApproachStep/um"() -> (w1062:dbl)
                          n237 = Wait (ms)(milliseconds to wait=u32 20) -> ()  [unwired: 1 out]
                          n238 = Number To Fractional String(number=w1062, precision (6)=i16 10) -> (F-format string=w1060:string)  [unwired: 2 in]
                          n239 = Concatenate Strings("MVR X " ("string"), w1060, "\n" ("string")) -> (w1057:string)
                          n240 = VISA Write(VISA resource name=w1068, write buffer=w1057, error in (no error)=w1067) -> (VISA resource name out=w1065:refnum<visa-resource-name>, error out=w1066:errorcluster)  [unwired: 1 out]
                          n241 = VISA Flush I/O Buffer(VISA resource name=w1065, error in (no error)=w1066) -> (VISA resource name out=w1064:refnum<visa-resource-name>, error out=w1063:errorcluster)  [unwired: 1 in]
                        }
                      }
                    }
                  }
                }
              }
            }
            n242 = Bundle(w876, w875) -> (→"XZ Graph":cluster{dbl[], dbl[]})  [unwired: 1 in]
          }
          frame #7 {
            n243 = local read "ColumnNum"() -> (w1084:i32)
            n244 = Equal?(x=w1088, y=0) -> (x = y?=w1092:bool)
            n245 = Decrement(x=w1084) -> (x-1=w1083:i32)
            n246 = Greater Or Equal?(x=w1090, y=w1083) -> (x >= y?=w1089:bool)
            n247 = case shown="True" w1092 {
              tunnel: w1090 -> [w1095 w1101]
              tunnel: w1091 -> [w1096 w1097]
              tunnel: [w1096 w1097] -> w1086
              tunnel: [w1095 w1101] -> w1085
              tunnel: w1089 -> [_ w1100]
              tunnel: w1088 -> [w1094 w1099]
              tunnel: [w1094 w1098] -> w1087
              frame False {
              }
              frame True {
                n248 = case shown="False" w1100 {
                  tunnel: w1099 -> [_ _]
                  tunnel: [1 -1] -> w1098
                  frame False {
                  }
                  frame True {
                  }
                }
              }
            }
          }
          frame #8 {
            n249 = Equal?(x=w1115, y=1) -> (x = y?=w1124:bool)
            n250 = Greater Or Equal?(x=w1105, y=w1116) -> (x >= y?=w1123:bool)
            n251 = And(x=w1124, y=w1123) -> (x .and. y?=w1122:bool)
            n252 = case shown="True" w1122 {
              tunnel: w1120 -> [w1127 w1131]
              tunnel: w1105 -> [w1126 w1129]
              tunnel: [w1127 w1130] -> w1119
              tunnel: [w1126 w1129] -> w1118
              tunnel: w1115 -> [w1125 _]
              tunnel: [w1125 0] -> w1117
              frame False {
              }
              frame True {
                n253 = Increment(x=w1131) -> (x+1=w1130:i32)
              }
            }
          }
          frame #9 {
            n254 = Equal?(x=w1148, y=-1) -> (x = y?=w1152:bool)
            n255 = Less Or Equal?(x=w1133, y=0) -> (x <= y?=w1150:bool)
            n256 = And(x=w1152, y=w1150) -> (x .and. y?=w1147:bool)
            n257 = case shown="True" w1147 {
              tunnel: w1148 -> [w1153 _]
              tunnel: w1146 -> [w1155 w1159]
              tunnel: w1133 -> [w1154 w1157]
              tunnel: [w1155 w1158] -> w1145
              tunnel: [w1154 w1157] -> w1144
              tunnel: [w1153 0] -> w1143
              frame False {
              }
              frame True {
                n258 = Increment(x=w1159) -> (x+1=w1158:i32)
              }
            }
          }
          frame #10 {
            n259 = Add(x=w1173, y=w1171) -> (x+y=w1170:i32)
          }
          frame #11 {
            n260 = local read "RowNum"() -> (w1185:i32)
            n261 = Greater Or Equal?(x=w1186, y=w1185) -> (x >= y?=w1184:bool)
          }
        }
        n262 = Compound Arithmetic op=OR(w427, w351) -> (w436:bool)
        "Counting" <- w357
      }
    }
    frame #6 {
      # "z"
      # "y"
      # "x"
      n263 = VISA Write(VISA resource name=w1199, write buffer="POS?\n", error in (no error)=w1198) -> (VISA resource name out=w1205:refnum<visa-resource-name>, error out=w1204:errorcluster)  [unwired: 1 out]
      n264 = VISA Read(VISA resource name=w1205, byte count=u32 128, error in (no error)=w1204) -> (VISA resource name out=w1197:refnum<visa-resource-name>, read buffer=w1201:string, error out=w1196:errorcluster)  [unwired: 1 out]
      n265 = Fract/Exp String To Number(string=w1201, offset=2) -> (number=w1195:dbl)  [unwired: 2 in, 1 out]
      n266 = local write "PIZPos"(w1195) -> ()
    }
    frame #7 {
    }
    frame #8 {
      n267 = VISA Write(VISA resource name=w1230, write buffer="MOV A 0\nMOV B 0\nERR?\n", error in (no error)=w1229) -> (VISA resource name out=w1227:refnum<visa-resource-name>, error out=w1226:errorcluster)  [unwired: 1 out]
      n268 = VISA Write(VISA resource name=w1222, write buffer="MOV X 0\n", error in (no error)=w1221) -> (VISA resource name out=w1220:refnum<visa-resource-name>, error out=w1219:errorcluster)  [unwired: 1 out]
      n269 = Wait (ms)(milliseconds to wait=u32 100) -> ()  [unwired: 1 out]
    }
  }
  n270 = VISA Write(VISA resource name=w25, write buffer="ERR?\n", error in (no error)=w24) -> (VISA resource name out=w23:refnum<visa-resource-name>, error out=w22:errorcluster)  [unwired: 1 out]
  n271 = local read "ColumnNum"() -> (w3:i32)
  n272 = VISA Close(VISA resource name=w43, error in (no error)=w42) -> ()  [unwired: 1 out]
  n273 = local read "RowNum"() -> (w4:i32)
  n274 = VISA Read(VISA resource name=w23, byte count=u32 128, error in (no error)=w22) -> (VISA resource name out=w21:refnum<visa-resource-name>, read buffer=w18:string, error out=w20:errorcluster)  [unwired: 1 out]
  n275 = call "Conversion.vi"("RowNum"=w4, "Y"=w29, "ComlNum"=w3, "X"=w28, "Z"=w27) -> ("YVector"=w2:dbl[], "XVector"=w1:dbl[], "ZMatrix"=w26:T1)
  n276 = local write "PIZERR? 2"(w18) -> ()
  n277 = VISA Close(VISA resource name=w41, error in (no error)=w40) -> ()  [unwired: 1 out]
  n278 = VISA Close(VISA resource name=w21, error in (no error)=w20) -> ()  [unwired: 1 out]
  n279 = call <vilib>:"create_plot_surface.vi"("z matrix"=w26, "y vector"=w2, "x vector"=w1) -> ("plots out"=→"3D Graph":refnum<class "Base Datatype.lvclass">[])  [unwired: 2 in, 6 out]
